vi "Ultrasonic.vi"(6 "Offset X":cluster{"Offset X L":dbl, "Offset X R":dbl}={"Offset X L"=15.0, "Offset X R"=15.0}, 8 "error in (no error)":errorcluster, 11 "Pulse in":T2) -> (0 "error out":errorcluster, 2 "PING":cluster{"PING left":dbl, "PING right":dbl}, 3 "Pulse out":T1)   [LabVIEW 2020]
uses:
  <vilib>/High Genius/HG_WSI_Tookit/Dependencies/Library/Pulse/Pulse.lvclass
  <vilib>/High Genius/HG_WSI_Tookit/Dependencies/Library/ISQ/ISQ.lvclass
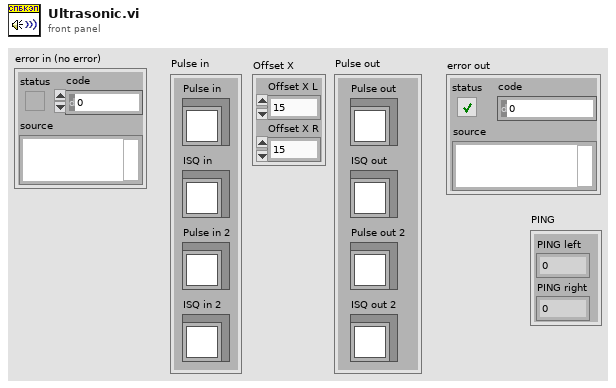
[diagram p1: front panel]
types:
  T1 = cluster{"Pulse out":refnum<class "Pulse.lvclass">, "ISQ out":refnum<class "ISQ.lvclass">, "Pulse out 2":refnum<class "Pulse.lvclass">, "ISQ out 2":refnum<class "ISQ.lvclass">}
  T2 = cluster{"Pulse in":refnum<class "Pulse.lvclass">, "ISQ in":refnum<class "ISQ.lvclass">, "Pulse in 2":refnum<class "Pulse.lvclass">, "ISQ in 2":refnum<class "ISQ.lvclass">}
  T3 = cluster{"Pulse out":refnum<class "Pulse.lvclass">, "ISQ out":refnum<class "ISQ.lvclass">, "Pulse out":refnum<class "Pulse.lvclass">, "ISQ out":refnum<class "ISQ.lvclass">}
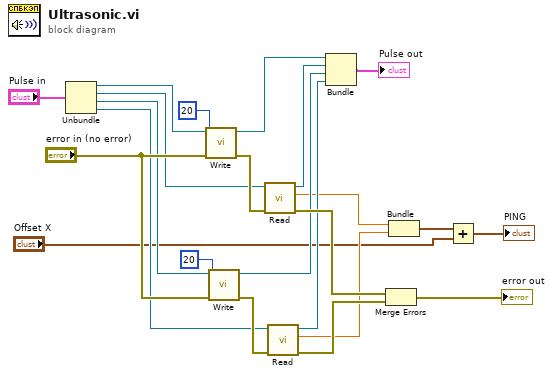
[diagram p0: block diagram]
diagram:
  n1 = Unbundle("Pulse in") -> ("Pulse in"=w11:refnum<class "Pulse.lvclass">, "ISQ in"=w12:refnum<class "ISQ.lvclass">, "Pulse in 2"=w13:refnum<class "Pulse.lvclass">, "ISQ in 2"=w14:refnum<class "ISQ.lvclass">)
  n2 = call <vilib>:"Write.vi"("error in (no error)"="error in (no error)", "Pulse"=20 ("Pluse"), "Pulse in"=w11) -> ("error out"=w22:errorcluster, "Pulse out"=w9:refnum<class "Pulse.lvclass">)  [unwired: 7 in]
  n3 = call <vilib>:"Write.vi"("error in (no error)"="error in (no error)", "Pulse"=20 ("Pluse"), "Pulse in"=w13) -> ("error out"=w20:errorcluster, "Pulse out"=w7:refnum<class "Pulse.lvclass">)  [unwired: 7 in]
  n4 = call <vilib>:"Read.vi"("error in (no error)"=w22, "ISQ in"=w12) -> ("error out"=w18:errorcluster, "PING"=w5:dbl, "ISQ out"=w8:refnum<class "ISQ.lvclass">)  [unwired: 7 in]
  n5 = call <vilib>:"Read.vi"("error in (no error)"=w20, "ISQ in"=w14) -> ("error out"=w17:errorcluster, "PING"=w4:dbl, "ISQ out"=w6:refnum<class "ISQ.lvclass">)  [unwired: 7 in]
  n6 = Bundle("Pulse out"=w9, "ISQ out"=w8, "Pulse out"=w7, "ISQ out"=w6) -> (→"Pulse out":T3)  [unwired: 1 in]
  n7 = Merge Errors(w18, w17) -> (→"error out":errorcluster)
  n8 = Bundle("PING"=w5, "PING"=w4) -> (w3:cluster{"PING":dbl, "PING":dbl})  [unwired: 1 in]
  n9 = Add(x=w3, y="Offset X") -> (x+y=→"PING":cluster{dbl, dbl})
